vi "Set Panel State.vi"(10 "Front Panel Window:State":T1(ring), 11 "Panel Open in":refnum<class "Base Queue.lvclass">) -> (3 "Panel Open out":refnum<class "Base Queue.lvclass">)   [LabVIEW 2021, in "jettl.lvlib" / "Base Queue.lvlib" / "Base Queue.lvclass"]
uses:
  Base Queue.lvclass
  Base Queue.lvclass/Base Queue.ctl
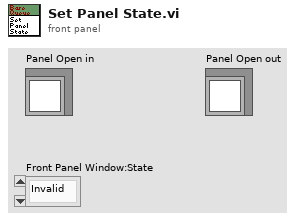
[diagram p1: front panel]
types:
  T1 = enum32{"Invalid", "Standard", "Closed", "Hidden", "Minimized", "Maximized"}
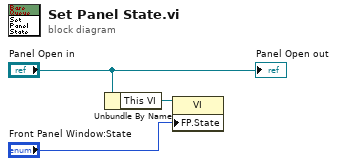
[diagram p0: block diagram]
diagram:
  n1 = Unbundle By Name("Panel Open in") -> ("This VI"=w3:refnum<vi>)
  n2 = property class="VI"(reference=w3, "FP.State"="Front Panel Window:State") -> ()  [unwired: 1 in, 2 out]
  "Panel Open out" <- "Panel Open in"
